vi "read png header.vi"() -> ()   [LabVIEW 2009]
uses:
  POLARIS Vision utility.lvlib
panel:
  out "Actual Index":i32
  out "error out":errorcluster
  out "string out":string
  out "header out":string
  in  "index (-1 last entry)":i32=-1
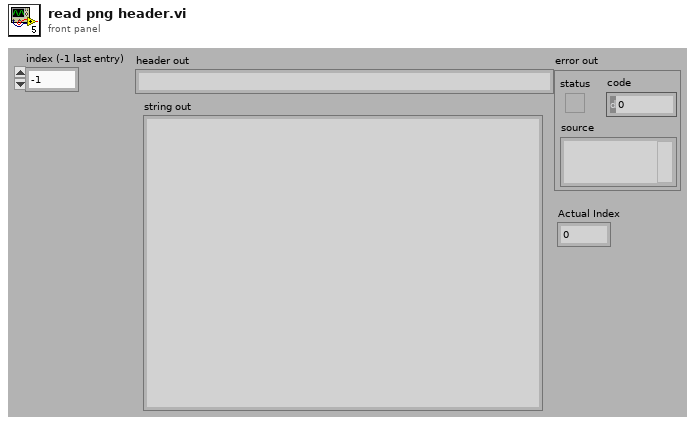
[diagram p1: front panel]
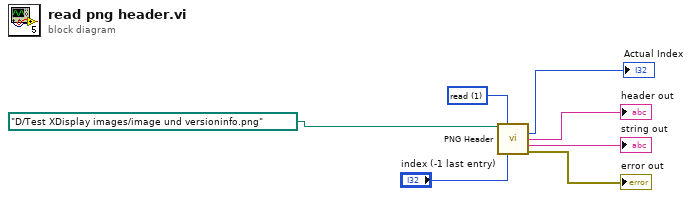
[diagram p0: block diagram]
diagram:
  w6 = u16 1 items=["Write", "read"] ("Mode")
  n1 = call "PNG Header.vi"("Path In"=path "D:/Test XDisplay images/image und versioninfo.png" ("File Path"), "Mode"=w6, "index (-1 last entry)"="index (-1 last entry)") -> ("Actual Index"=→"Actual Index":i32, "header out"=→"header out":string, "string out"=→"string out":string, "error out"=→"error out":errorcluster)  [unwired: 8 in, 1 out]
